vi "Counter Close.vi"(8 "error in":errorcluster, 11 "couner session in":T1) -> (0 "error out":errorcluster, 3 "counter session out":T1)   [LabVIEW 2018, in "Counter.lvlib"]
doc: "Closes counter session."
uses:
  Counter.lvlib
  Counter Session.ctl
  Counter Type.ctl
  <vilib>/Instr/_visa.llb/VISA GPIB Control REN Mode.ctl
  Picotest U62XXA/PICOTEST U62XXA series.lvlib
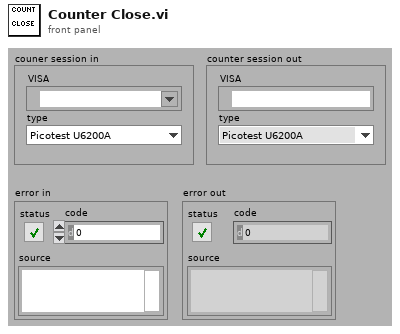
[diagram p1: front panel]
types:
  T1 = typedef "Counter.lvlib/Counter Session.ctl" = cluster{"VISA":refnum<visa-resource-name>, "type":T2}
  T2 = typedef "Counter.lvlib/Counter Type.ctl" = enum16{"Picotest U6200A", "dummy"}
  T3 = typedef "VISA GPIB Control REN Mode.ctl" = u16
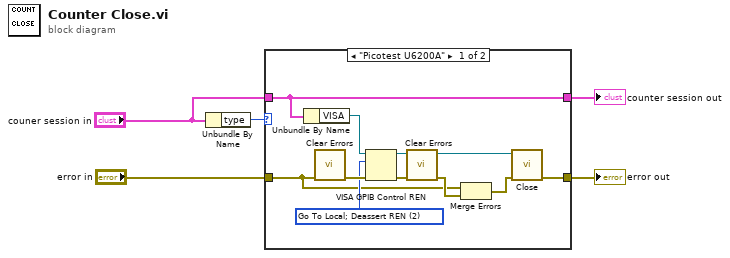
[diagram p0: block diagram]
diagram:
  n1 = Unbundle By Name("couner session in") -> ("type"=w5:T2)
  n2 = case shown="\"Picotest U6200A\"" w5 {
    tunnel: "error in" -> [w7 w17]
    tunnel: "couner session in" -> [w14 w16]
    tunnel: [w15 w17] -> w3
    tunnel: [w14 w16] -> w1
    frame "Picotest U6200A" {
      w11 = T3 2 items=["Deassert REN", "Assert REN", "Go To Local; Deassert REN ", "Assert REN; Address Device", "Local Lockout (Addressed Devices)", "Local Lockout (This Device)", "Go To Local"] ("Mode")
      n3 = Unbundle By Name(w14) -> ("VISA"=w12:refnum<visa-resource-name>)
      n4 = call <vilib>:"Clear Errors.vi"("error in (no error)"=w7) -> ("error out"=w13:errorcluster)  [unwired: 5 in, 1 out]
      n5 = VISA GPIB Control REN(8:w13, 10:w11, 11:w12) -> (0:w10:errorcluster, 3:w9:refnum<visa-resource-name>)
      n6 = call <vilib>:"Clear Errors.vi"("error in (no error)"=w10) -> ("error out"=w8:errorcluster)  [unwired: 5 in, 1 out]
      n7 = Merge Errors(w7, w8) -> (w6:errorcluster)
      n8 = call "Close.vi"("error in (no error)"=w6, "VISA resource name"=w9) -> ("error out"=w15:errorcluster)  [unwired: 9 in]
    }
    frame Default {
    }
  }
  "error out" <- w3
  "counter session out" <- w1
